vi "DatabaseAPI-Delete.vi"(7 "Where Statement":string, 8 "error in (no error)":errorcluster, 10 "table":string, 11 "Database-API in":refnum<class "Database-API.lvclass">) -> (0 "error out":errorcluster, 3 "Database-API out":refnum<class "Database-API.lvclass">)   [LabVIEW 2014, in "Database-API.lvclass"]
uses:
  Database-API.lvclass
  Database-API.lvclass/Database-API.ctl
  <vilib>/addons/database/NI_Database_API.lvlib
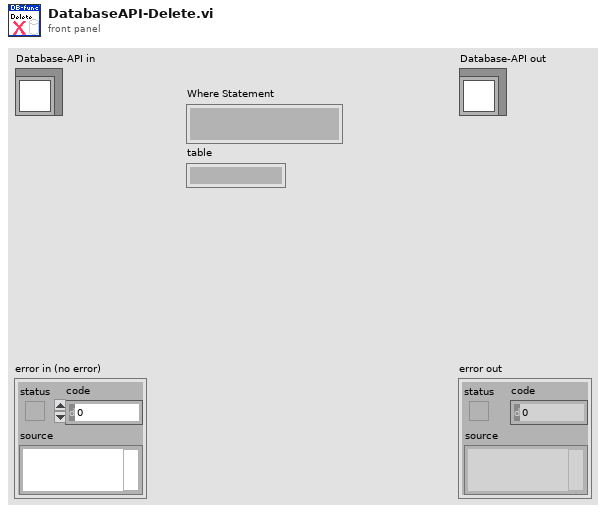
[diagram p1: front panel]
types:
  T1 = typedef "NI_Database_API.lvlib/Conn ObjectReference.ctl" = refnum<k1>
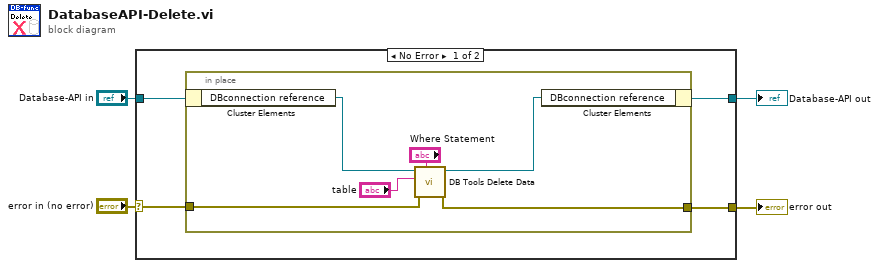
[diagram p0: block diagram]
diagram:
  n1 = case shown="No Error" "error in (no error)" {
    selector: "error in (no error)" -> [w7 w16]
    tunnel: [w6 w16] -> w3
    tunnel: [w5 w15] -> w1
    tunnel: "Database-API in" -> [w8 w15]
    frame No Error {
      n2 = in-place {
        in-place-border: w7 -> [w10]
        in-place-border: [w9] -> w6
        n3 = in-place-cluster #1(w8) -> ("DBconnection reference"=w13:T1)
        n4 = call <vilib>:"DB Tools Delete Data.vi"("condition"="Where Statement", "error in (no error)"=w10, "table"="table", "connection reference"=w13) -> ("error out"=w9:errorcluster, "connection reference out"=w12:T1)  [unwired: 6 in]
        n5 = in-place-cluster #1("DBconnection reference"=w12) -> (w5:refnum<class "Database-API.lvclass">)
      }
    }
    frame Error {
    }
  }
  "error out" <- w3
  "Database-API out" <- w1
